vi "conversion_pos_in_lab.vi"(3 "error in (no error)":errorcluster caption="错误输入（无错误）", 4 "pos":dbl, 5 "OneMotion 输入":refnum<class "OneMotion.lvclass">) -> (0 "error out":errorcluster caption="错误输出", 1 "pos in lab":dbl, 2 "OneMotion 输出":refnum<class "OneMotion.lvclass">)   [LabVIEW 2016, in "MotionControl.lvlib" / "OneMotion.lvclass"]
uses:
  <userlib>/MotionControl/OneMotion/OneMotion.lvclass
  <userlib>/MotionControl/OneMotion/OneMotion.lvclass/OneMotion.ctl
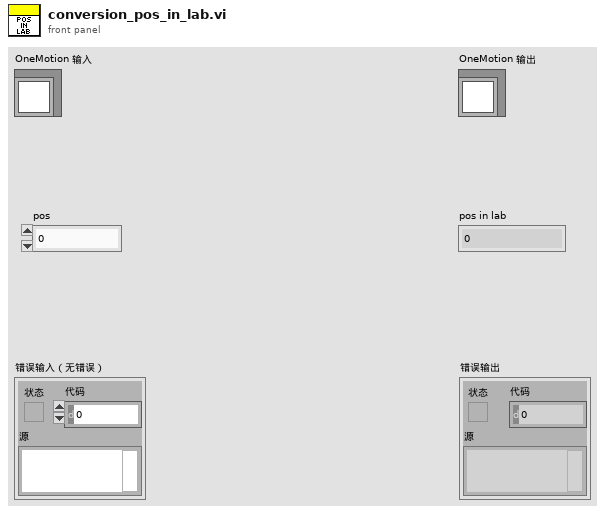
[diagram p1: front panel]
types:
  T1 = typedef "MotionControl.lvlib/OneMotion.lvclass/unit mode.ctl" = enum16{"motor (pulse)", "linear (mm) or radial (degree)"}
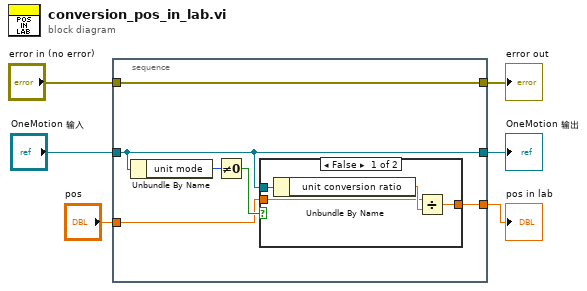
[diagram p0: block diagram]
diagram:
  n1 = stacked-sequence {
    tunnel: [w12] -> w6
    tunnel: [w7] -> w4
    tunnel: "OneMotion 输入" -> [w7]
    tunnel: "pos" -> [w9]
    tunnel: [w8] -> w2
    tunnel: "error in (no error)" -> [w12]
    frame #0 {
      n2 = Unbundle By Name(w7) -> ("unit mode"=w11:T1)
      n3 = Not Equal To 0?(x=w11) -> (x != 0?=w10:bool)
      n4 = case shown="False" w10 {
        tunnel: w9 -> [w15 w17]
        tunnel: [w14 w17] -> w8
        tunnel: w7 -> [w13 _]
        frame False {
          n5 = Unbundle By Name(w13) -> ("unit conversion ratio"=w16:dbl)
          n6 = Divide(x=w15, y=w16) -> (x/y=w14:dbl)
        }
        frame True {
        }
      }
    }
  }
  "error out" <- w6
  "OneMotion 输出" <- w4
  "pos in lab" <- w2
